vi "LiftClose.vi"   [LabVIEW 2014, in "LiftLib.lvlib"]
uses:
  LiftLib.lvlib
  LiftRefs.ctl
types:
  T1 = typedef "LiftLib.lvlib/LiftRefs.ctl" = enum16{"LiftCim1", "LiftCim2", "LiftEncoder", "LiftLimitSwitch1", "LiftLimitSwitch2"}
  T2 = typedef "WPI_MotorControlDeviceRef.ctl" = cluster{"DeviceStatus":errorcluster, "Type":T3, "PWM":cluster{"Controller":T4, "PWM Channel":T5, "DeadBand":T6}, "CAN":cluster{"Device Number":u8, "Control Mode":T7, "Semaphore":T8, "Max Vout":dbl, "TalonSRX Control Mode":T9}, "Invert":bool, "TransformRef":T10, "InvTransformRef":T10}
  T3 = typedef "WPI_MotorControlType.ctl" = enum16{"PWM", "CAN", "CANTalonSRX"}
  T4 = typedef "FPGA_TypedefDigitalModule.ctl" = enum16{"Controller 1"}
  T5 = typedef "FPGA_DIOPWMChannel.ctl" = enum8{"PWM 0", "PWM 1", "PWM 2", "PWM 3", "PWM 4", "PWM 5", "PWM 6", "PWM 7", "PWM 8", "PWM 9", "PWM MXP 0", "PWM MXP 1", "PWM MXP 2", "PWM MXP 3", "PWM MXP 4", "PWM MXP 5", "PWM MXP 6", "PWM MXP 7", "PWM MXP 8", "PWM MXP 9", "Invalid"}
  T6 = typedef "WPI_PWMDeadband.ctl" = cluster{"Name":string, "maxPositivePwm":i32, "minPositivePwm":i32, "centerPwm":i32, "maxNegativePwm":i32, "minNegativePwm":i32, "angularRange":u16}
  T7 = typedef "WPI_CANJaguar_ControlMode.ctl" = enum8{"Percent VBus", "Current", "Speed", "Position", "Voltage"}
  T8 = typedef "Semaphore RefNum" = refnum<k1>
  T9 = typedef "WPI_CANTalonSRX_APIControlMode.ctl" = enum8{"Percent VBus", "Speed", "Position", "Slave", "Unchanged / Invalid"}
  T10 = typedef "WPI_PWMTransform_ConPane.ctl" = refnum<vi>
  T11 = typedef "WPI_EncoderDevRef.ctl" = cluster{"DevStatus":errorcluster, "EncoderIndex":T12, "CounterIndex":T13, "DistancePerCount":dbl, "Decoding Type":T14}
  T12 = typedef "FPGA_EncoderIdx.ctl" = enum8{"Enc 0", "Enc 1", "Enc 2", "Enc 3", "Enc 4", "Enc 5", "Enc 6", "Enc 7", "Invalid"}
  T13 = typedef "FPGA_CounterCtrSystemIndex.ctl" = enum8{"Ctr 0", "Ctr 1", "Ctr 2", "Ctr 3", "Ctr 4", "Ctr 5", "Ctr 6", "Ctr 7", "Invalid"}
  T14 = typedef "WPI_EncoderType.ctl" = enum16{"1x", "2x", "4x"}
  T15 = typedef "WPI_DigitalInputDevRef.ctl" = cluster{"DevStatus":errorcluster, "DIO Channel":T16, "Controller":T4}
  T16 = typedef "FPGA_DIOChannel.ctl" = enum8{"DIO 0", "DIO 1", "DIO 2", "DIO 3", "DIO 4", "DIO 5", "DIO 6", "DIO 7", "DIO 8", "DIO 9", "DIO MXP 0", "DIO MXP 1", "DIO MXP 2", "DIO MXP 3", "DIO MXP 4", "DIO MXP 5", "DIO MXP 6", "DIO MXP 7", "DIO MXP 8", "DIO MXP 9", "DIO MXP 10", "DIO MXP 11", "DIO MXP 12", "DIO MXP 13", "DIO MXP 14", "DIO MXP 15", "Invalid"}
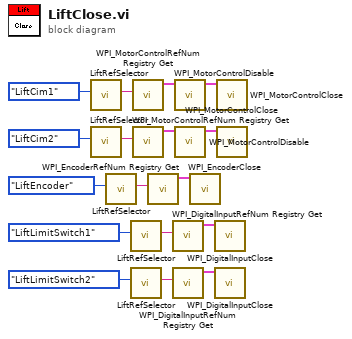
[diagram p0: block diagram]
diagram:
  n1 = call "LiftRefSelector.vi"("LiftRefs"=LiftRefs."LiftCim1") -> ("String"=w16:string)  [unwired: 10 in]
  n2 = call "LiftRefSelector.vi"("LiftRefs"=LiftRefs."LiftCim2") -> ("String"=w12:string)  [unwired: 10 in]
  n3 = call "LiftRefSelector.vi"("LiftRefs"=LiftRefs."LiftEncoder") -> ("String"=w7:string)  [unwired: 10 in]
  n4 = call "LiftRefSelector.vi"("LiftRefs"=LiftRefs."LiftLimitSwitch1") -> ("String"=w4:string)  [unwired: 10 in]
  n5 = call "LiftRefSelector.vi"("LiftRefs"=LiftRefs."LiftLimitSwitch2") -> ("String"=w3:string)  [unwired: 10 in]
  n6 = call <vilib>:"WPI_MotorControlRefNum Registry Get.vi"("refnum name"=w16) -> ("MotorControlDevRef"=w15:T2)  [unwired: 9 in, 1 out]
  n7 = call <vilib>:"WPI_MotorControlRefNum Registry Get.vi"("refnum name"=w12) -> ("MotorControlDevRef"=w11:T2)  [unwired: 9 in, 1 out]
  n8 = call <vilib>:"WPI_EncoderRefNum Registry Get.vi"("refnum name"=w7) -> ("EncoderDevRef"=w9:T11)  [unwired: 9 in, 1 out]
  n9 = call <vilib>:"WPI_DigitalInputRefNum Registry Get.vi"("refnum name"=w4) -> ("DigitalInputDevRef"=w2:T15)  [unwired: 9 in, 1 out]
  n10 = call <vilib>:"WPI_DigitalInputRefNum Registry Get.vi"("refnum name"=w3) -> ("DigitalInputDevRef"=w1:T15)  [unwired: 9 in, 1 out]
  n11 = call <vilib>:"WPI_MotorControlDisable.vi"("MotorControlDevRef"=w15) -> ("MotorControlDevRef"=w14:T2)  [unwired: 9 in, 1 out]
  n12 = call <vilib>:"WPI_MotorControlDisable.vi"("MotorControlDevRef"=w11) -> ("MotorControlDevRef"=w10:T2)  [unwired: 9 in, 1 out]
  n13 = call <vilib>:"WPI_EncoderClose.vi"("EncoderDevRef"=w9) -> ()  [unwired: 10 in, 1 out]
  n14 = call <vilib>:"WPI_DigitalInputClose.vi"("DigitalInputDevRef"=w2) -> ()  [unwired: 10 in, 1 out]
  n15 = call <vilib>:"WPI_DigitalInputClose.vi"("DigitalInputDevRef"=w1) -> ()  [unwired: 10 in, 1 out]
  n16 = call <vilib>:"WPI_MotorControlClose.vi"("MotorControlDevRef"=w14) -> ()  [unwired: 10 in, 1 out]
  n17 = call <vilib>:"WPI_MotorControlClose.vi"("MotorControlDevRef"=w10) -> ()  [unwired: 10 in, 1 out]
